vi "Engine.vi"(7 "Action":T2, 8 "error in (no error)":errorcluster, 11 "Variant in":variant) -> (0 "error out":errorcluster, 3 "Variant out":variant)   [LabVIEW 2018, in "Help.lvlib"]
uses:
  Help.lvlib
  Action.ctl
panel:
  in  "StateData":T1
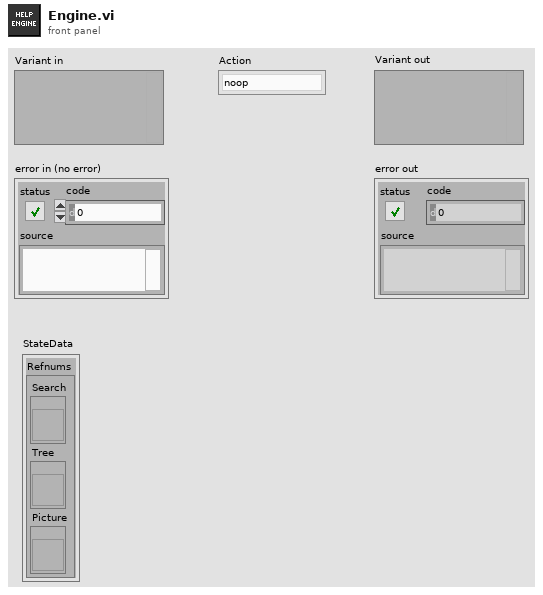
[diagram p1: front panel]
types:
  T1 = cluster{"Refnums":cluster{"Search":refnum<vi>, "Tree":refnum<vi>, "Picture":refnum<vi>}}
  T2 = typedef "Help.lvlib/Action.ctl" = enum8{"noop", "new", "init", "close", "load", "render", "filter", "topic"}
  T3 = cluster{"Search":refnum<vi>, "Tree":refnum<vi>, "Picture":refnum<vi>}
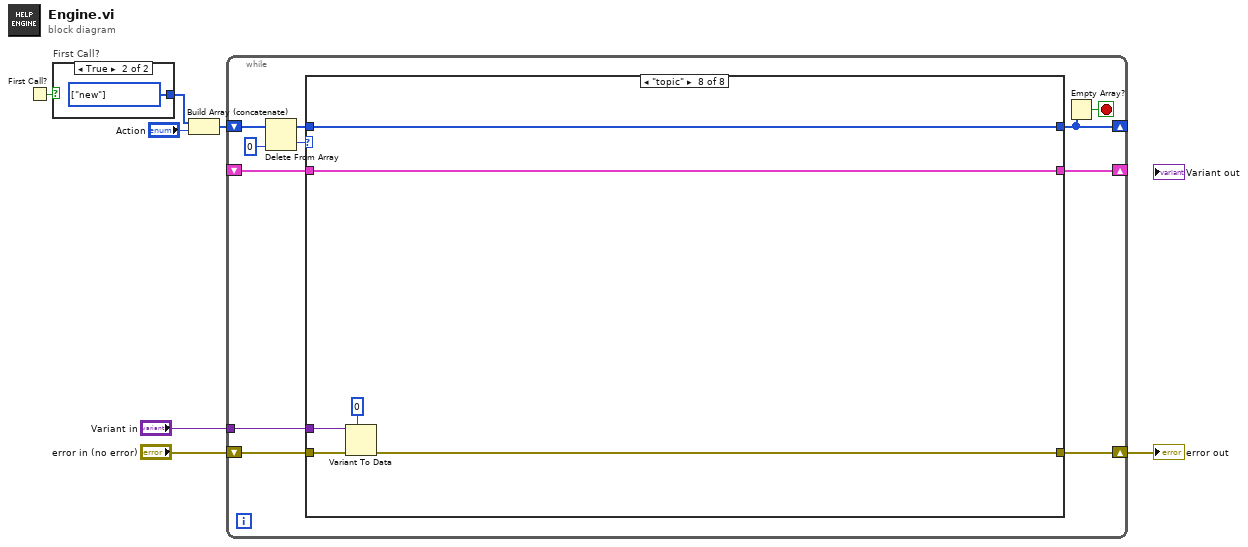
[diagram p0: block diagram]
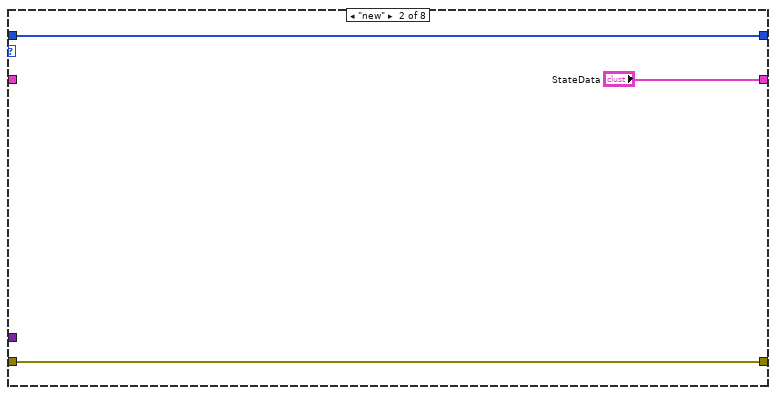
[diagram p3: hidden frame]
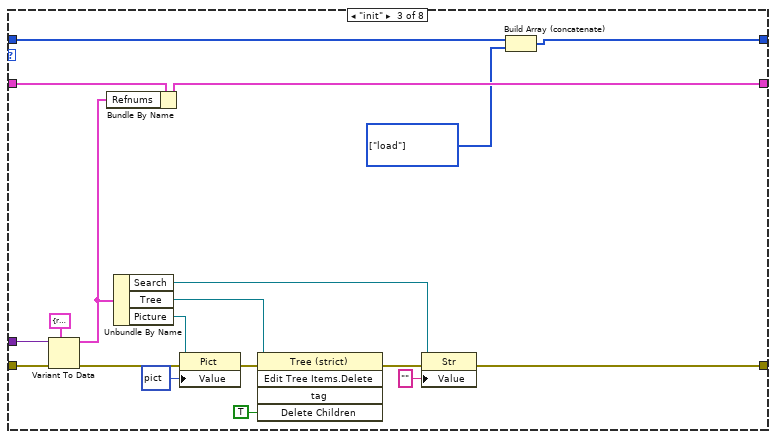
[diagram p4: hidden frame]
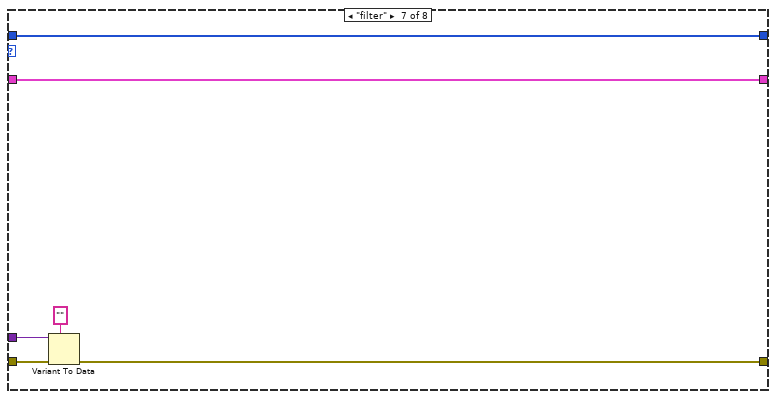
[diagram p8: hidden frame]
diagram:
  n1 = First Call?() -> (First Call?: T/F=w2:bool)
  n2 = case "First Call?" shown="True" w2 {
    tunnel: [_ w8] -> w1
    frame False {
    }
    frame True {
      w8 = T2[] [enum."new"] items=["noop", "new", "init", "close", "load", "render", "filter", "topic"] ("appended array")
    }
  }
  n3 = Build Array (concatenate)(w1, "Action") -> (w6:T2[])
  n4 = while {
    shift-right: [w13] -> _
    shift-left: w6 -> [w19]
    shift-right: [w14] -> w4
    shift-left: "error in (no error)" -> [w15]
    tunnel: "Variant in" -> [w11]
    shift-right: [w10] -> _
    shift-left: _ -> [w9]
    stop <- w12 stop-if-true
    n5 = Delete From Array(array=w19, index=0) -> (deleted portion=w17:T2, array with subset deleted=w16:T2[])  [unwired: 1 in]
    n6 = case shown="\"topic\"" w17 {
      tunnel: [w22 w25 w27 w47 w50 w53 w59 w65] -> w13
      tunnel: w16 -> [w22 w25 w44 w47 w50 w53 w59 w65]
      tunnel: w15 -> [w21 w24 w43 w46 w49 w52 w58 w64]
      tunnel: [w21 w24 w32 w46 w49 w52 w57 w63] -> w14
      tunnel: w11 -> [_ _ w41 _ _ _ w56 w62]
      tunnel: [w20 "StateData" w29 w45 w48 w51 w54 w61] -> w10
      tunnel: w9 -> [w20 _ w39 w45 w48 w51 w54 w61]
      frame "noop", Default {
      }
      frame "new" {
      }
      frame "init" {
        w26 = T2[] [enum."load"] items=["noop", "new", "init", "close", "load", "render", "filter", "topic"] ("array")
        n7 = Variant To Data(error in=w43, type=T3 {"Search"=refnum, "Tree"=refnum, "Picture"=refnum} ("Init"), Variant=w41) -> (data=w28:T3, error out=w42:errorcluster)
        n8 = Bundle By Name(cluster=w39, "Refnums"=w28) -> (w29:T1)
        n9 = Unbundle By Name(w28) -> ("Search"=w31:refnum<vi>, "Tree"=w34:refnum<vi>, "Picture"=w37:refnum<vi>)
        n10 = property class="Pict"(reference=w37, error in=w42, "Value"=picture data[5B]) -> (error out=w38:errorcluster)  [unwired: 1 out]
        n11 = invoke class="Tree (strict)" method="Edit Tree Items.Delete"(reference=w34, error in=w38, "Delete Children"=TRUE ("Delete Children?")) -> (error out=w35:errorcluster)  [unwired: 2 in, 4 out]
        n12 = property class="Str"(reference=w31, error in=w35, "Value"="") -> (error out=w32:errorcluster)  [unwired: 1 out]
        n13 = Build Array (concatenate)(w44, w26) -> (w27:T2[])
      }
      frame "close" {
      }
      frame "load" {
      }
      frame "render" {
      }
      frame "filter" {
        n14 = Variant To Data(error in=w58, type="", Variant=w56) -> (error out=w57:errorcluster)  [unwired: 1 out]
      }
      frame "topic" {
        n15 = Variant To Data(error in=w64, type=0, Variant=w62) -> (error out=w63:errorcluster)  [unwired: 1 out]
      }
    }
    n16 = Empty Array?(array=w13) -> (empty?=w12:bool)
  }
  "error out" <- w4
